vi "ProyectoBioCuinique Early Acces.vi"() -> ()   [LabVIEW 2021]
uses:
  <vilib>/Utility/NIReport.llb/Report Type.ctl
  <extravilib>/ChannelInstances/Tag-dbl/Read With Abort.vi
  <extravilib>/ChannelInstances/Tag-bool/Read With Abort.vi
  <extravilib>/ChannelInstances/Tag-bool/Write With Abort.vi
  <extravilib>/ChannelInstances/Tag-dbl/Write With Abort.vi
  <vilib>/Instr/_visa.llb/VISA Configure Serial Port (Instr).vi
  <vilib>/MakerHub/LINX/Public/Utilities/Open Serial.vi
  <extravilib>/ChannelInstances/Tag-dbl/Instantiate.vi
  <extravilib>/ChannelInstances/Tag-bool/Instantiate.vi
  <extravilib>/ChannelInstances/Tag-dbl/EndpointRead.vi
  <vilib>/addons/_office/excel.llb/Excel Easy Table (str).vi
  <extravilib>/ChannelInstances/Tag-bool/EndpointRead.vi
  <extravilib>/ChannelInstances/Tag-bool/Endpoint.vi
  <extravilib>/ChannelInstances/Tag-dbl/Endpoint.vi
  <vilib>/Utility/NIReport.llb/NI_report.lvclass
  <vilib>/LabVIEW Interface for Arduino/LabVIEW Interface for Arduino.lvlib
  <vilib>/MakerHub/LINX/LMH-LINX.lvlib
  <vilib>/Utility/NIReport.llb/NI_ReportGenerationCore.lvlib
  <vilib>/addons/_office/NI_ReportGenerationToolkit.lvlib
  <vilib>/Utility/NIReport.llb/Excel/NI_Excel.lvclass
  <vilib>/MakerHub/LINX/Public/Sensors/Distance/Ultrasonic/Ultrasonic.lvlib
  <extravilib>/ChannelInstances/Tag-bool.lvlib
  <extravilib>/ChannelInstances/Tag-dbl.lvlib
panel:
  out "?":dbl
  out "Hs2 4/3":dbl(knob) scale=0.0..100.0
  out "?":dbl
  out "Hs2 4/2":dbl(knob) scale=0.0..100.0
  out "?":dbl
  out "Hs2 3/3 2":dbl(knob) scale=0.0..100.0
  out "?":dbl
  out "Hs2 3/2":dbl(knob) scale=0.0..100.0
  out "?":dbl
  out "?":dbl
  out "Hs2 2/3":dbl(knob) scale=0.0..100.0
  out "Hs2 2/2":dbl(knob) scale=0.0..100.0
  out "?":dbl
  out "Hs2/3":dbl(knob) scale=0.0..100.0
  out "?":dbl
  out "Hs2/2":dbl(knob) scale=0.0..100.0
  out "Hs2 4/1":dbl(knob) scale=0.0..100.0
  out "C° 4":dbl(slide) scale=0.0..50.0
  out "?":dbl
  out "?":dbl
  out "?":dbl
  out "Hr1 4":dbl(knob) scale=0.0..100.0
  out "Hs2 3/1":dbl(knob) scale=0.0..100.0
  out "C° 3":dbl(slide) scale=0.0..50.0
  out "?":dbl
  out "?":dbl
  out "?":dbl
  out "Hr1 3":dbl(knob) scale=0.0..100.0
  out "Hs2 2/1":dbl(knob) scale=0.0..100.0
  out "C° 2":dbl(slide) scale=0.0..50.0
  out "?":dbl
  out "?":dbl
  out "?":dbl
  out "Hr1 2":dbl(knob) scale=0.0..100.0
  out "cm 2":dbl
  out "Nivel de Agua 2":dbl(slide) scale=0.0..275.0
  out "Nivel de Agua":dbl(slide) scale=0.0..275.0
  in  "?":u8
  in  "?":u8
  in  "?":u8
  out "?":bool
  in  "?":bool
  out "?":bool
  in  "?":bool
  out "?":bool
  out "Hs2/1":dbl(knob) scale=0.0..100.0
  out "C°":dbl(slide) scale=0.0..50.0
  out "?":dbl
  in  "ARDUINO\nDE SENSORES\nULTRASÓNICOS":refnum<visa-resource-name>="N/A"
  in  "DATOS \n      DE  REGISTRO":path
  in  "?":u8
  in  "?":u8
  in  "?":u8
  out "?":dbl
  in  "ARDUINO DE \nSENSORES Y HUMEDAD \nY TEMPERATURA":refnum<visa-resource-name>
  out "?":dbl
  out "Hr1":dbl(knob) scale=0.0..100.0
  out "cm":dbl
  out "?":bool
  in  "?":bool
  out "?":bool
  in  "?":bool
  out "?":bool
  in  "?":bool
  in  "ARDUINO DE \nVÁLVULAS":refnum<visa-resource-name>
  # "BOMBA 1"
  # "VÁLVULA 1"
  # "VÁLVULA 2"
  # "VÁLVULA 3"
  # "BOMBA 2"
  # "VÁLVULA 4"
  # "SENSORES LINEA 2"
  # "SENSORES LINEA 4"
  # "SENSORES LINEA 1"
  # "SENSORES LINEA 3"
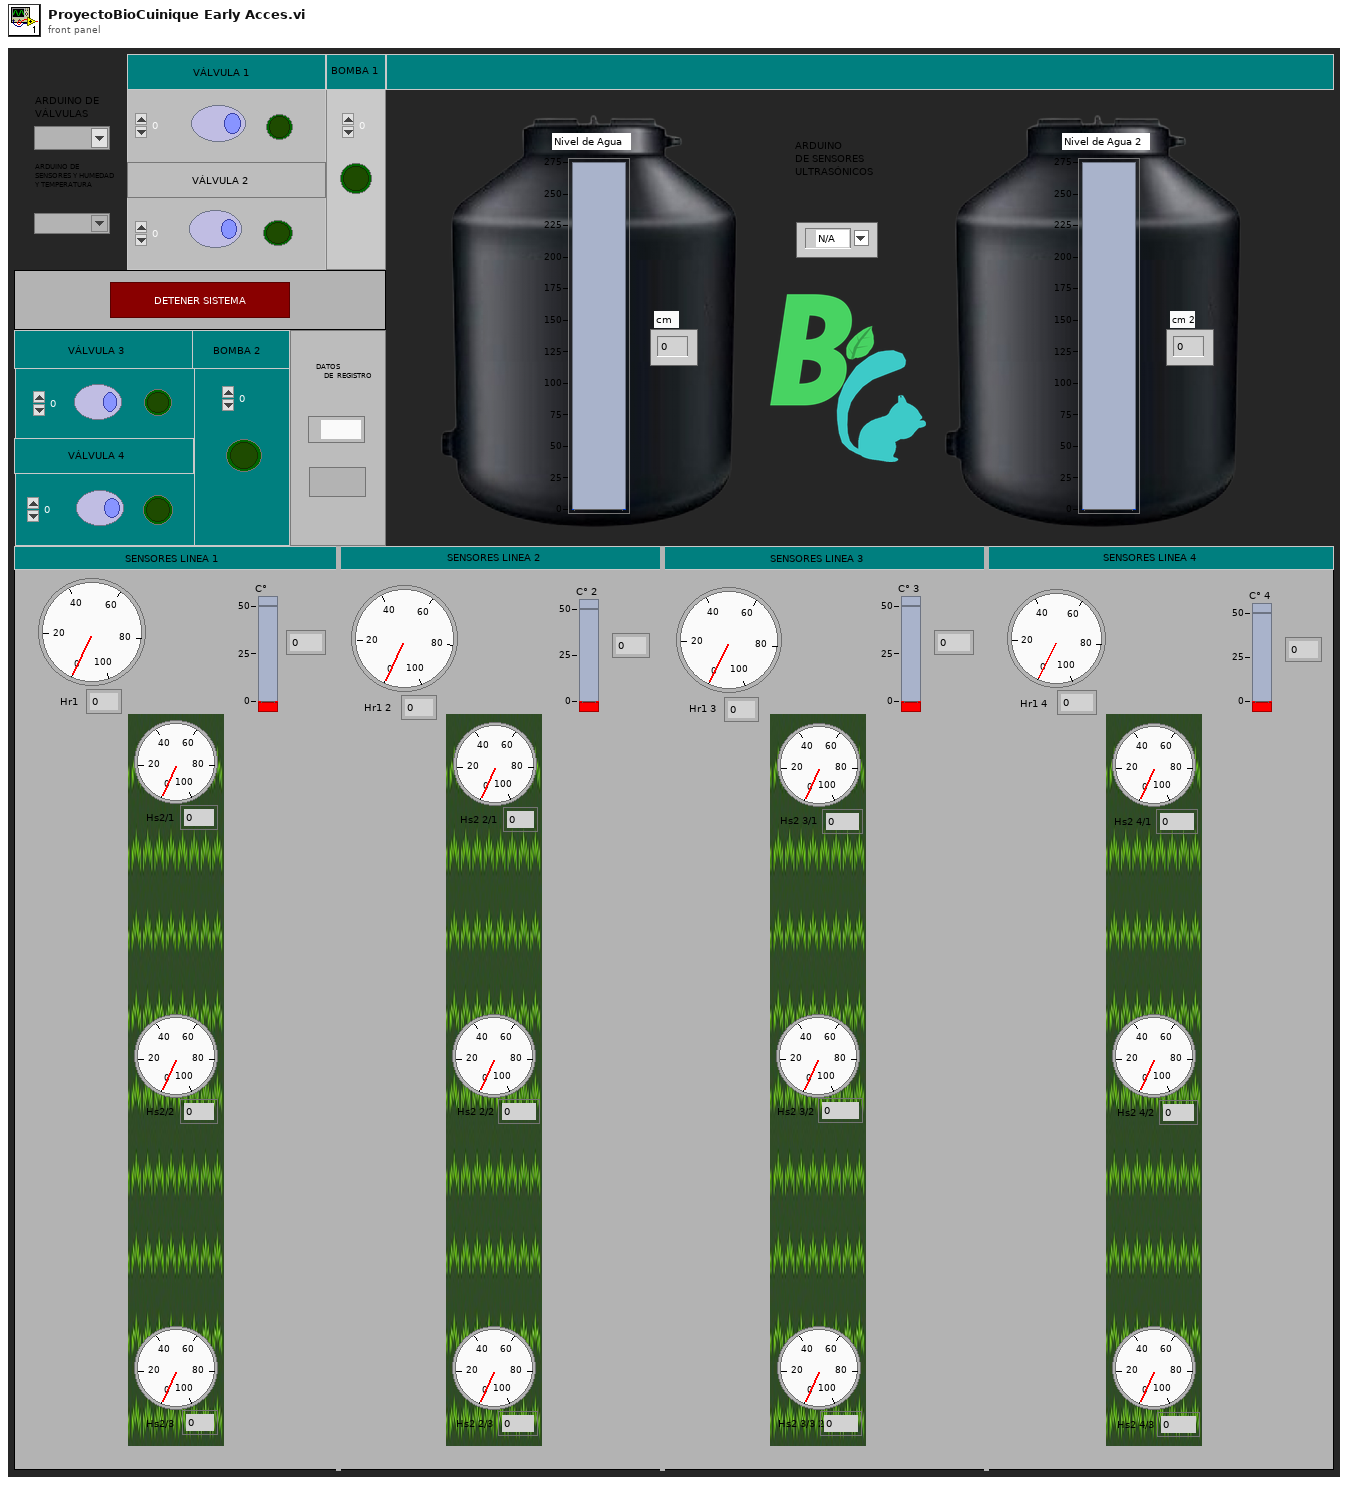
[diagram p1: front panel]
types:
  T1 = typedef "NI_ReportGenerationCore.lvlib/Report Type.ctl" = enum16{"HTML", "Word", "Excel"}
  T2 = typedef "LMH-LINX.lvlib/LINX Ref.ctl" = cluster{"IO":T3, "Interface":T4, "LINX Device Config":T5}
  T3 = typedef "LMH-LINX.lvlib/Platform.ctl" = enum16{"Remote", "Local"}
  T4 = typedef "LMH-LINX.lvlib/Interface.ctl" = enum16{"Serial", "TCP"}
  T5 = typedef "LMH-LINX.lvlib/Device.lvlib/LINX Device Config.ctl" = cluster{"Interface":T4, "COM Port":refnum<visa-resource-name>, "TCP Configuration":T6, "Device Family":u8, "Device ID":u8, "Device Name":string, "TCP Ref":refnum<k5>, "Channels":T7}
  T6 = typedef "LMH-LINX.lvlib/Device.lvlib/TCP Config.ctl" = cluster{"IP Address":string, "Port":u16}
  T7 = typedef "LMH-LINX.lvlib/Channels.ctl" = cluster{"DI":u8[], "DO":u8[], "AI":u8[], "AO":u8[], "PWM":u8[], "QE":u8[], "UART":u8[], "I2C 2":u8[], "SPI":u8[], "CAN":u8[], "Servo":u8[], "AI Ref (V)":dbl, "AI Resolution (Bits)":u8, "AO Ref (V)":dbl, "AO Resolution (Bits)":u8}
  T8 = typedef "LabVIEW Interface for Arduino.lvlib/Arduino Resource.ctl" = cluster{"VISA resource":refnum<visa-resource-name>, "Board Type":T9, "Connection Type":enum8{"USB / Serial"}, "Bytes Per Packet (15)":u8}
  T9 = typedef "LabVIEW Interface for Arduino.lvlib/Board Type.ctl" = enum16{"Uno", "Dimuelanove w/Atmega 328", "Mega 2560"}
  T10 = typedef "Tag-bool.lvlib/))Channel.ctl" = refnum<queue>
  T11 = typedef "Tag-dbl.lvlib/))Channel.ctl" = refnum<queue>
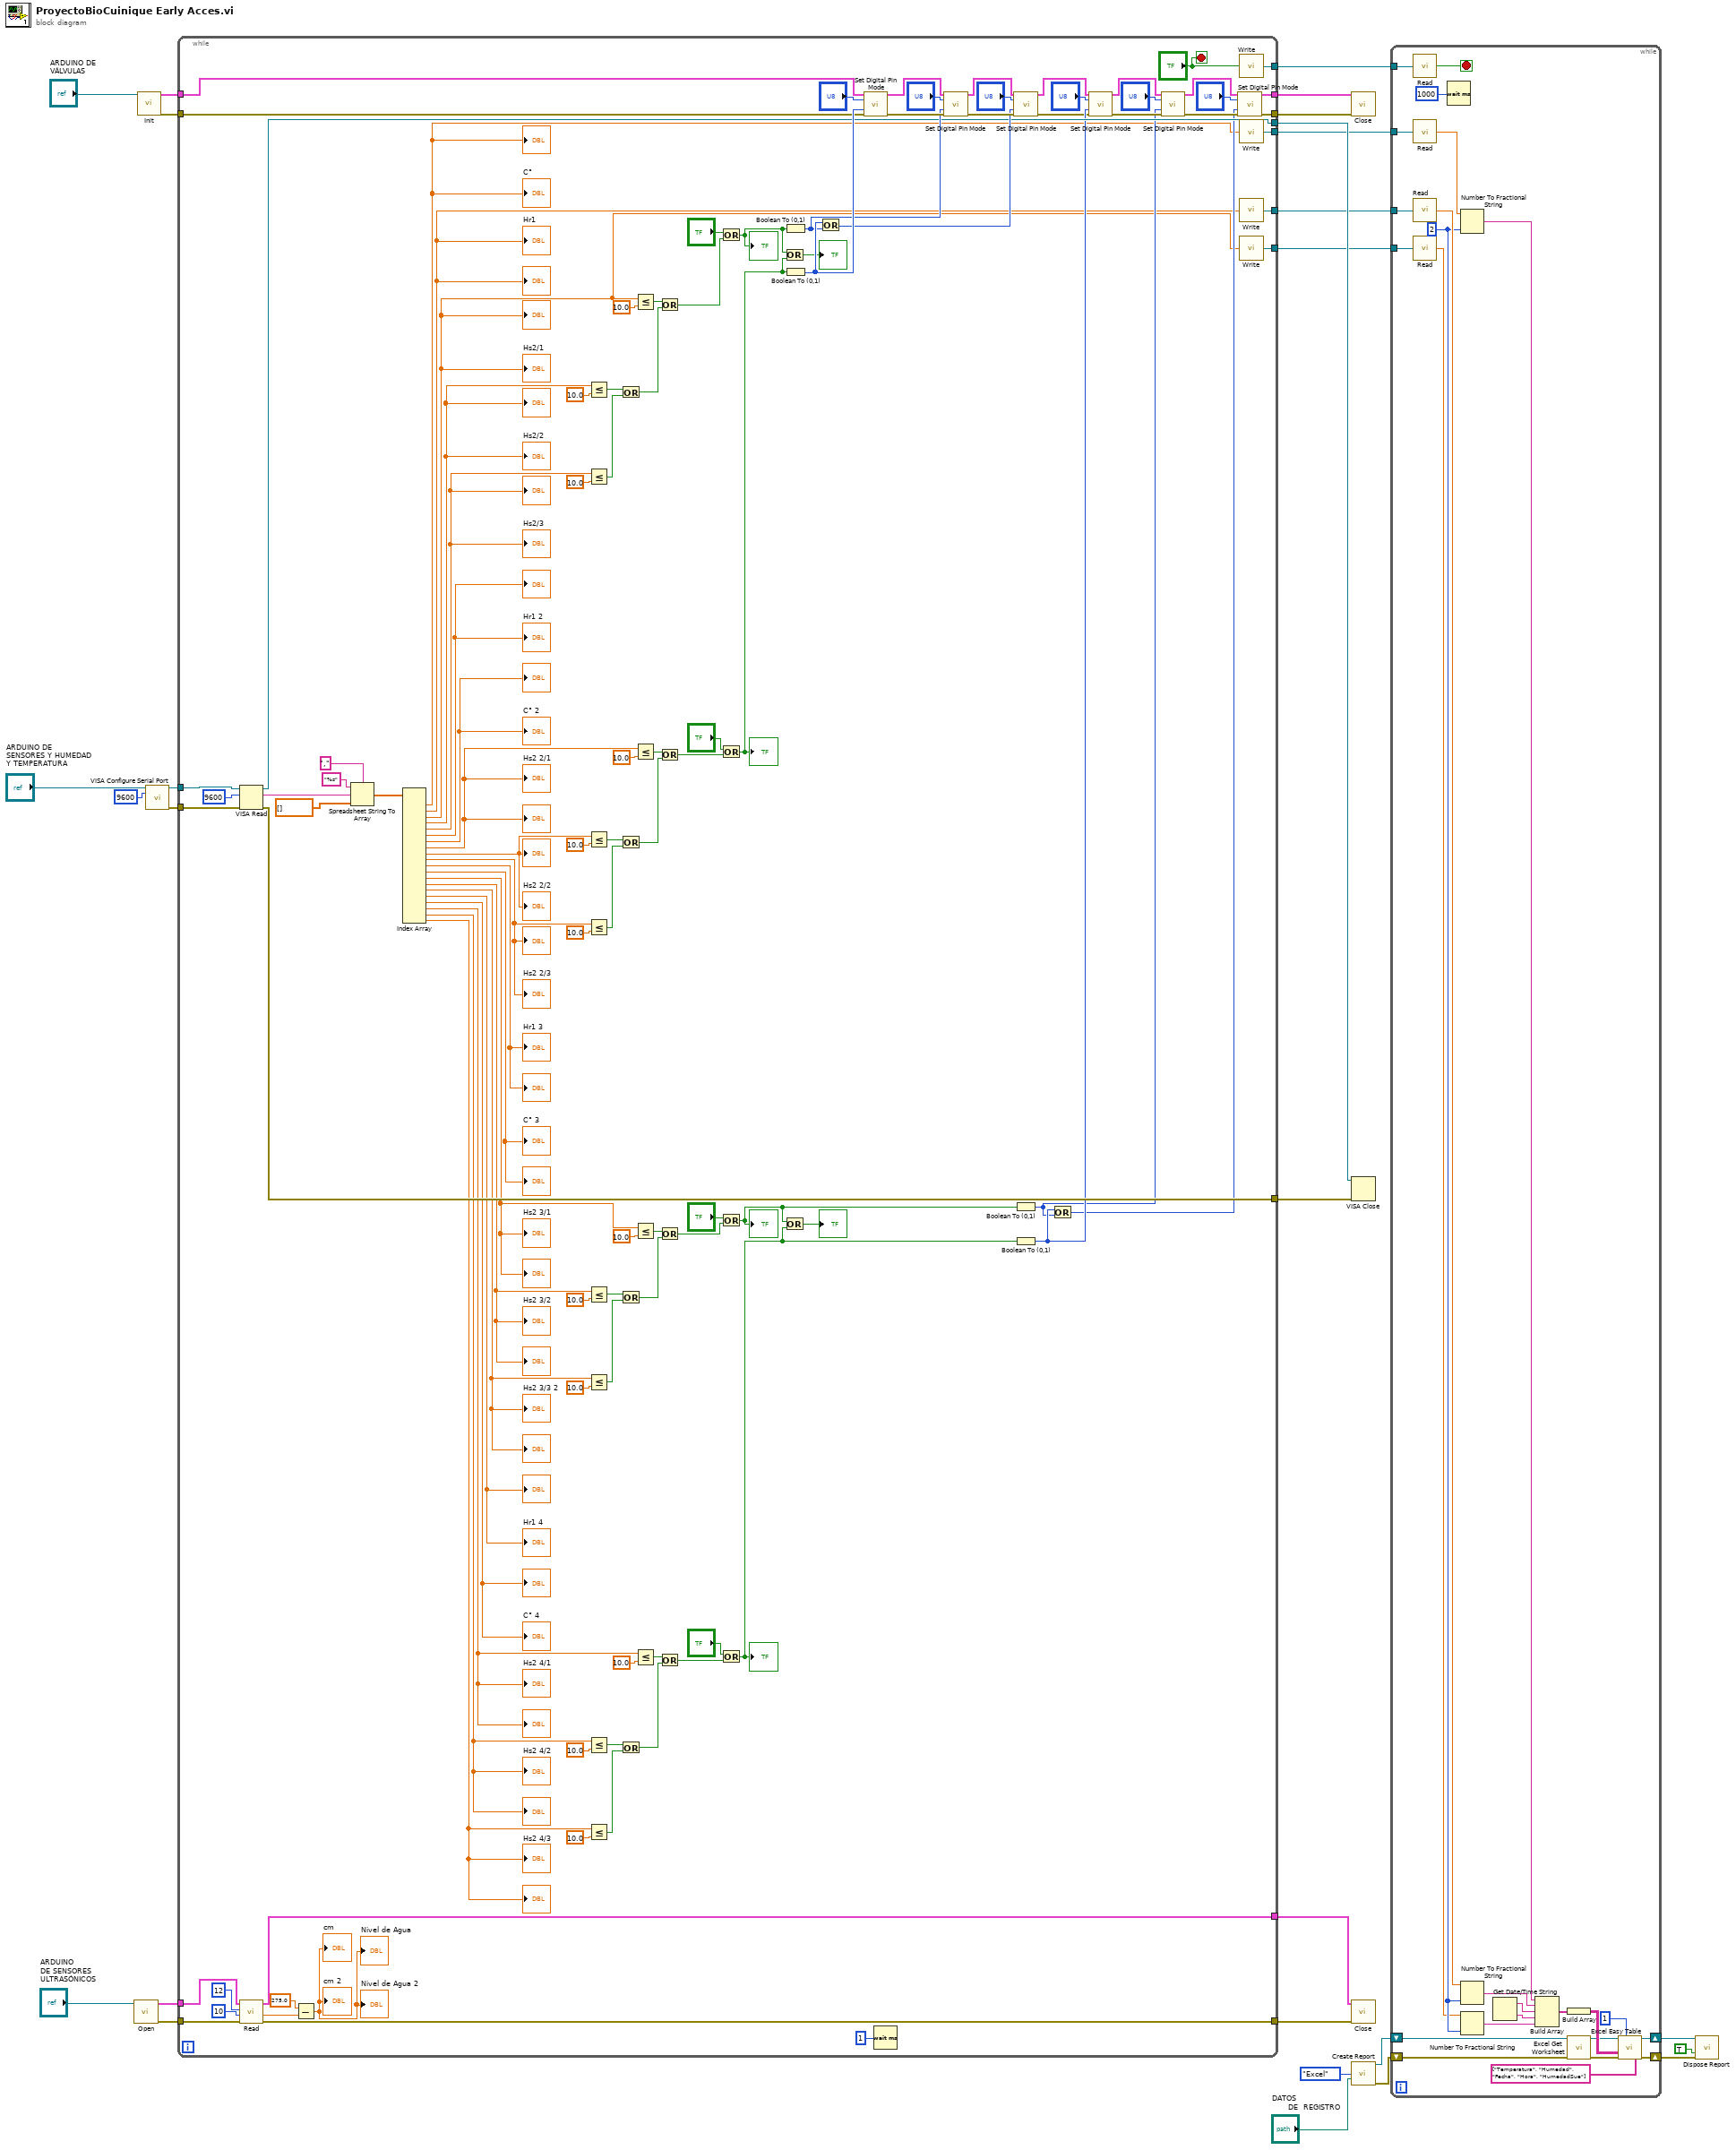
[diagram p0: block diagram]
diagram:
  n1 = call-poly <vilib>:"Open.vi"("Serial Port"="ARDUINO\nDE SENSORES\nULTRASÓNICOS") -> ("Error Out"=w26:errorcluster, "LINX Resource"=w25:T2)  [unwired: 8 in, 1 out]
  n2 = call <vilib>:"Init.vi"("VISA resource"="ARDUINO DE \nVÁLVULAS") -> ("Arduino Resource"=w4:T8, "error out"=w3:errorcluster)  [unwired: 17 in]
  n3 = call-poly "VISA Configure Serial Port"("VISA resource name"="ARDUINO DE \nSENSORES Y HUMEDAD \nY TEMPERATURA", "baud rate (9600)"=u32 9600) -> ("VISA resource name out"=w22:refnum<visa-resource-name>, "error out"=w19:errorcluster)  [unwired: 12 in]
  n4 = while {
    tunnel: w26 -> [w128]
    tunnel: w25 -> [w129]
    tunnel: [w127] -> w24
    tunnel: [w126] -> w23
    tunnel: w22 -> [w125]
    tunnel: [w124] -> w21
    tunnel: [w123] -> w20
    tunnel: w19 -> [w122]
    tunnel: [w108] -> w9
    tunnel: [w107] -> w8
    tunnel: [w106] -> w7
    tunnel: [w103] -> w5
    tunnel: w4 -> [w84]
    tunnel: w3 -> [w83]
    tunnel: [w82] -> w2
    tunnel: [w81] -> w1
    stop <- "?" stop-if-true
    n5 = VISA Read(VISA resource name=w125, byte count=u32 9600, error in (no error)=w122) -> (VISA resource name out=w123:refnum<visa-resource-name>, read buffer=w121:string, error out=w124:errorcluster)  [unwired: 1 out]
    n6 = call <vilib>:"Read.vi"("Error In"=w128, "DO Channel"=u8 10, "DI Channel"=u8 12, "LINX Resource"=w129) -> ("Error Out"=w126:errorcluster, "Centimeters"=w80:dbl, "LINX Resource"=w127:T2)  [unwired: 4 in, 1 out]
    n7 = Subtract(x=275.0, y=w80) -> (x-y=→"cm" →"Nivel de Agua" →"Nivel de Agua 2" →"cm 2":dbl)
    n8 = Spreadsheet String To Array(delimiter (Tab)=",", format string="%s", spreadsheet string=w121, array type (2D Dbl)=dbl[] []) -> (array=w117:dbl[])
    n9 = Index Array(array=w117) -> (element #1=w68:dbl, element #2=w72:dbl, element #3=w71:dbl, element #4=w62:dbl, element #5=w60:dbl, element #6=→"Hr1 2" →"?":dbl, element #7=→"C° 2" →"?":dbl, element #8=w66:dbl, element #9=w47:dbl, element #10=w46:dbl, element #11=→"?" →"Hr1 3":dbl, element #12=→"?" →"C° 3":dbl, element #13=w65:dbl, element #14=w38:dbl, element #15=w37:dbl, element #16=→"Hr1 4" →"?":dbl, element #17=→"C° 4" →"?":dbl, element #18=w64:dbl, element #19=w29:dbl, element #20=w28:dbl)  [unwired: 20 in]
    "Hr1" <- w72
    "?" <- w68
    "?" <- w72
    "?" <- w71
    "C°" <- w68
    "Hs2/1" <- w71
    "?" <- w65
    "Hs2 3/1" <- w65
    "Hs2 4/1" <- w64
    "Hs2 2/1" <- w66
    "?" <- w64
    "?" <- w66
    "Hs2 3/3 2" <- w37
    "?" <- w37
    "Hs2/2" <- w62
    "?" <- w62
    "Hs2/3" <- w60
    "?" <- w60
    "Hs2 2/2" <- w47
    "Hs2 2/3" <- w46
    "?" <- w46
    "?" <- w47
    "Hs2 3/2" <- w38
    "?" <- w38
    "Hs2 4/2" <- w29
    "?" <- w29
    "Hs2 4/3" <- w28
    "?" <- w28
    n10 = Less Or Equal?(x=w62, y=10.0) -> (x <= y?=w58:bool)
    n11 = Less Or Equal?(x=w60, y=10.0) -> (x <= y?=w59:bool)
    n12 = Less Or Equal?(x=w47, y=10.0) -> (x <= y?=w51:bool)
    n13 = Less Or Equal?(x=w46, y=10.0) -> (x <= y?=w52:bool)
    n14 = Less Or Equal?(x=w38, y=10.0) -> (x <= y?=w42:bool)
    n15 = Less Or Equal?(x=w37, y=10.0) -> (x <= y?=w43:bool)
    n16 = Less Or Equal?(x=w29, y=10.0) -> (x <= y?=w33:bool)
    n17 = Less Or Equal?(x=w28, y=10.0) -> (x <= y?=w34:bool)
    n18 = Or(x=w58, y=w59) -> (x .or. y?=w57:bool)
    n19 = Or(x=w51, y=w52) -> (x .or. y?=w50:bool)
    n20 = Or(x=w42, y=w43) -> (x .or. y?=w41:bool)
    n21 = Or(x=w33, y=w34) -> (x .or. y?=w32:bool)
    n22 = Less Or Equal?(x=w71, y=10.0) -> (x <= y?=w56:bool)
    n23 = Less Or Equal?(x=w66, y=10.0) -> (x <= y?=w49:bool)
    n24 = Less Or Equal?(x=w65, y=10.0) -> (x <= y?=w40:bool)
    n25 = Less Or Equal?(x=w64, y=10.0) -> (x <= y?=w31:bool)
    n26 = Or(x=w56, y=w57) -> (x .or. y?=w55:bool)
    n27 = Or(x=w49, y=w50) -> (x .or. y?=w48:bool)
    n28 = Or(x=w40, y=w41) -> (x .or. y?=w39:bool)
    n29 = Or(x=w31, y=w32) -> (x .or. y?=w30:bool)
    n30 = Or(x="?", y=w55) -> (x .or. y?=w113:bool)
    "?" <- w113
    n31 = Or(x="?", y=w48) -> (x .or. y?=w104:bool)
    "?" <- w104
    n32 = Or(x="?", y=w39) -> (x .or. y?=w93:bool)
    "?" <- w93
    n33 = Or(x="?", y=w30) -> (x .or. y?=w88:bool)
    "?" <- w88
    n34 = Or(x=w113, y=w104) -> (x .or. y?=→"?":bool)
    n35 = Or(x=w93, y=w88) -> (x .or. y?=→"?":bool)
    n36 = Boolean To (0,1)(Boolean=w113) -> (0, 1=w135:i16)
    n37 = Boolean To (0,1)(Boolean=w104) -> (0, 1=w136:i16)
    n38 = Or(x=w136, y=w135) -> (x .or. y?=w134:i16)
    n39 = call <vilib>:"Set Digital Pin Mode.vi"("Arduino Resource"=w84, "Digital I/O Pin"="?", "Pin Mode (Input)"=w136, "error in"=w83) -> ("Arduino Resource"=w140:T8, "error out"=w139:errorcluster)  [unwired: 10 in]
    n40 = Wait (ms)(milliseconds to wait=u32 1) -> ()  [unwired: 1 out]
    n41 = call <vilib>:"Set Digital Pin Mode.vi"("Arduino Resource"=w140, "Digital I/O Pin"="?", "Pin Mode (Input)"=w135, "error in"=w139) -> ("Arduino Resource"=w137:T8, "error out"=w138:errorcluster)  [unwired: 10 in]
    n42 = call <vilib>:"Set Digital Pin Mode.vi"("Arduino Resource"=w137, "Digital I/O Pin"="?", "Pin Mode (Input)"=w134, "error in"=w138) -> ("Arduino Resource"=w87:T8, "error out"=w86:errorcluster)  [unwired: 10 in]
    n43 = Boolean To (0,1)(Boolean=w93) -> (0, 1=w97:i16)
    n44 = Boolean To (0,1)(Boolean=w88) -> (0, 1=w98:i16)
    n45 = Or(x=w98, y=w97) -> (x .or. y?=w96:i16)
    n46 = call <vilib>:"Set Digital Pin Mode.vi"("Arduino Resource"=w87, "Digital I/O Pin"="?", "Pin Mode (Input)"=w98, "error in"=w86) -> ("Arduino Resource"=w102:T8, "error out"=w101:errorcluster)  [unwired: 10 in]
    n47 = call <vilib>:"Set Digital Pin Mode.vi"("Arduino Resource"=w102, "Digital I/O Pin"="?", "Pin Mode (Input)"=w97, "error in"=w101) -> ("Arduino Resource"=w99:T8, "error out"=w100:errorcluster)  [unwired: 10 in]
    n48 = call <vilib>:"Set Digital Pin Mode.vi"("Arduino Resource"=w99, "Digital I/O Pin"="?", "Pin Mode (Input)"=w96, "error in"=w100) -> ("Arduino Resource"=w82:T8, "error out"=w81:errorcluster)  [unwired: 10 in]
    n49 = call <extravilib>:"Write.vi"("element"="?") -> ("channel"=w108:T10)  [unwired: 1 out]
    n50 = call <extravilib>:"Write.vi"("element"=w68) -> ("channel"=w107:T11)  [unwired: 1 out]
    n51 = call <extravilib>:"Write.vi"("element"=w72) -> ("channel"=w106:T11)  [unwired: 1 out]
    n52 = call <extravilib>:"Write.vi"("element"=w71) -> ("channel"=w103:T11)  [unwired: 1 out]
  }
  n53 = call <vilib>:"Close.vi"("Arduino Resource"=w2, "error in"=w1) -> ()  [unwired: 13 in, 1 out]
  n54 = VISA Close(VISA resource name=w20, error in (no error)=w21) -> ()  [unwired: 1 out]
  n55 = call <vilib>:"Close.vi"("Error In"=w23, "LINX Resource"=w24) -> ()  [unwired: 9 in, 1 out]
  n56 = call <vilib>:"Create Report.vi"("report type"=Report_Type."Excel", "template (empty)"="DATOS \n      DE  REGISTRO") -> ("report out"=w13:refnum<class "NI_report.lvclass">, "error out"=w14:errorcluster)  [unwired: 12 in]
  n57 = while {
    shift-right: [w154] -> w11
    shift-left: w14 -> [w159]
    shift-right: [w155] -> w12
    shift-left: w13 -> [w157]
    tunnel: w9 -> [w150]
    tunnel: w8 -> [w148]
    tunnel: w7 -> [w146]
    tunnel: w5 -> [w144]
    stop <- w149 stop-if-true
    w143 = i16 2 ("precision (6)")
    n58 = call <vilib>:"Read.vi"("channel"=w150) -> ("element"=w149:bool)  [unwired: 1 in, 1 out]
    n59 = call <vilib>:"Read.vi"("channel"=w148) -> ("element"=w147:dbl)  [unwired: 1 in, 1 out]
    n60 = call <vilib>:"Read.vi"("channel"=w146) -> ("element"=w145:dbl)  [unwired: 1 in, 1 out]
    n61 = call <vilib>:"Read.vi"("channel"=w144) -> ("element"=w142:dbl)  [unwired: 1 in, 1 out]
    n62 = Wait (ms)(milliseconds to wait=u32 1000) -> ()  [unwired: 1 out]
    n63 = Number To Fractional String(number=w147, precision (6)=w143) -> (F-format string=w165:string)  [unwired: 2 in]
    n64 = Number To Fractional String(number=w145, precision (6)=w143) -> (F-format string=w164:string)  [unwired: 2 in]
    n65 = Number To Fractional String(number=w142, precision (6)=w143) -> (F-format string=w141:string)  [unwired: 2 in]
    n66 = Get Date/Time String() -> (date string=w163:string, time string=w162:string)  [unwired: 3 in]
    n67 = Build Array(w165, w164, w163, w162, w141) -> (w161:string[])
    n68 = Build Array(w161) -> (w160:string[][])
    n69 = call <vilib>:"Excel Get Worksheet.vi"("report in"=w157, "error in (no error)"=w159) -> ("report out"=w156:refnum<class "NI_report.lvclass">, "error out"=w158:errorcluster)  [unwired: 12 in]
    n70 = call-poly <vilib>:"Excel Easy Table.vi"("report in"=w156, "iteration"=1, "text data"=w160, "error in (no error)"=w158, "column headers"=string[] ["Temperatura", "Humedad", "Fecha", "Hora", "HumedadSue"]) -> ("report out"=w155:refnum<class "NI_report.lvclass">, "error out"=w154:errorcluster)  [unwired: 6 in, 3 out]
  }
  n71 = call-dynamic "Dispose Report.vi"("report in"=w12, "save changes? (F)"=TRUE, "error in (no error)"=w11) -> ()  [unwired: 12 in, 1 out]
